vi "avaliaPresoNaParede.vi"(10 "Robot in":T3, 11 "IA State":T2={"our_robots"=[], "enemy_robots"=[], "balls"=[], "geometry"={"field_length"=0, "field_width"=0, "goal_width"=0, "goal_depth"=0, "center_circle_radius"=0, "defense_width"=0, "defense_depth"=0, "free_kick_from_defense_dist"=0, "penalty_spot_from_field_line_dist"=0, "penalty_line_from_spot_dist"=0, "half_moon_depth"=0, "half_moon_width"=0}, "IA Judge"={"stage"="", "command"="", "our_goalie_id"=0.0, "enemy_goalie_id"=0.0, "command enum"=enum."Halt", "Time"=enum."Azul"}, "Received Timestamp"=timestamp(0 s since 1904-01-01), "Events"={"Touch"=FALSE, "id touch"=0.0, "Ball out of \nVision"=FALSE, "Ball inside \nGoalie area"=FALSE, "Robot not responding"=FALSE, "Robots responding status"=[1.0, 1.0, 1.0, 1.0, 1.0, 1.0], "Enemy Ball \nPossession"=FALSE, "Id ini Possession"=0.0, "Ball Possesion"=FALSE, "Id Possesion"=0.0, "Ball at\nour goal side"=FALSE, "Ball at\ntouchline"=FALSE, "Ball at\nenemy goal side"=FALSE}}) -> (2 "Parede":T1(ring), 3 "Preso na parede?":bool=TRUE)   [LabVIEW 2018]
uses:
  Intel/Functions Enum.ctl
  Intel/AttackerStates.ctl
  Path Planning/RRT/PathDest.ctl
  Path Planning/RRT/PathDests.ctl
  Core/AI Robot.ctl
  Core/AI Ball.ctl
  Core/Field Size.ctl
  Intel/Command Enum.ctl
  Core/AI Judge.ctl
  Util/Events/Events.ctl
  Core/AI Input.ctl
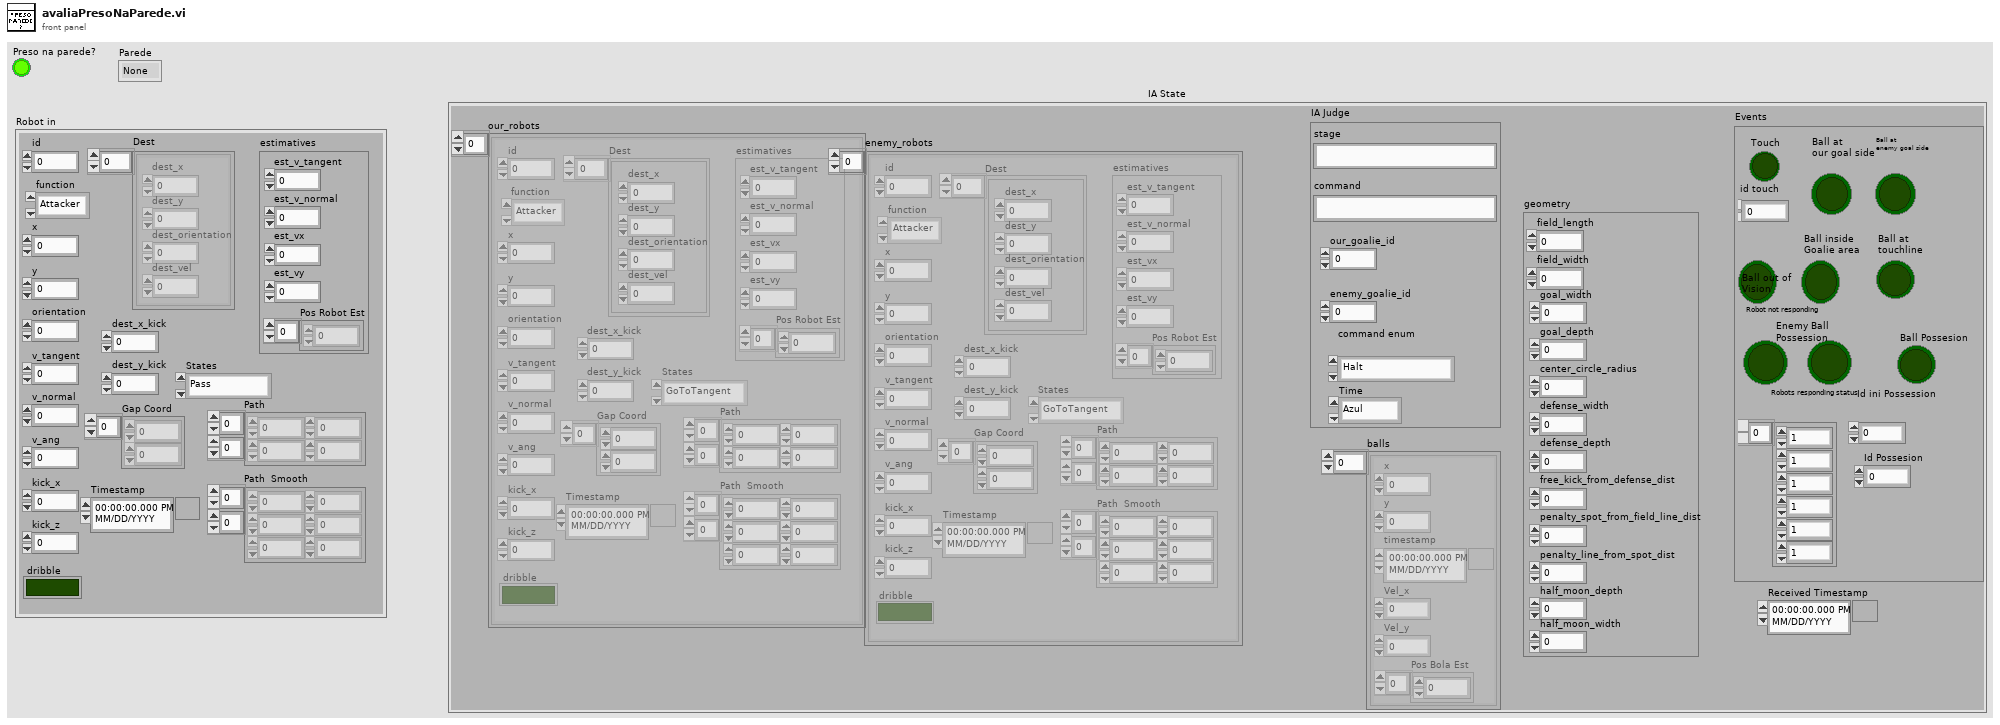
[diagram p1: front panel]
types:
  T1 = enum16{"None", "Frente", "Trás", "Cima", "Baixo"}
  T2 = typedef "AI Input.ctl" = cluster{"our_robots":T3[], "enemy_robots":T3[], "balls":T8[], "geometry":T9, "IA Judge":T10, "Received Timestamp":timestamp, "Events":T12}
  T3 = typedef "AI Robot.ctl" = cluster{"id":u32, "function":T4, "x":dbl, "y":dbl, "orientation":dbl, "v_tangent":dbl, "v_normal":dbl, "v_ang":dbl, "kick_x":dbl, "kick_z":dbl, "dribble":bool, "Timestamp":timestamp, "estimatives":cluster{"est_v_tangent":dbl, "est_v_normal":dbl, "est_vx":dbl, "est_vy":dbl, "Pos Robot Est":dbl[]}, "dest_x_kick":dbl, "dest_y_kick":dbl, "Gap Coord":dbl[], "States":T5, "Path ":dbl[][], "Path  Smooth":dbl[][], "Dest":T6}
  T4 = typedef "Functions Enum.ctl" = enum16{"Attacker", "Goalie", "Defender", "Striker", "Goto 0", "Dummy", "Kicker", "ZigZag"}
  T5 = typedef "AttackerStates.ctl" = enum16{"Pass", "GoToTangent", "BallGetting", "GoToKick", "Rotate anti-clockwise", "Rotate Clockwise", ""}
  T6 = typedef "PathDests.ctl" = T7[]
  T7 = typedef "PathDest.ctl" = cluster{"dest_x":dbl, "dest_y":dbl, "dest_orientation":dbl, "dest_vel":dbl}
  T8 = typedef "AI Ball.ctl" = cluster{"x":dbl, "y":dbl, "timestamp":timestamp, "Vel_x":dbl, "Vel_y":dbl, "Pos Bola Est":dbl[]}
  T9 = typedef "Field Size.ctl" = cluster{"field_length":u32, "field_width":u32, "goal_width":u32, "goal_depth":u32, "center_circle_radius":u32, "defense_width":u32, "defense_depth":u32, "free_kick_from_defense_dist":u32, "penalty_spot_from_field_line_dist":u32, "penalty_line_from_spot_dist":u32, "half_moon_depth":u32, "half_moon_width":u32}
  T10 = typedef "AI Judge.ctl" = cluster{"stage":string, "command":string, "our_goalie_id":dbl, "enemy_goalie_id":dbl, "command enum":T11, "Time":enum16{"Azul", "Amarelo"}}
  T11 = typedef "Command Enum.ctl" = enum16{"Halt", "Stop", "Force Start", "PKA Normal Start", "Prepare Kickoff Ally", "PKE Normal Start", "Prepare Kickoff Enemy", "Prepare Penalty Ally", "PPA Normal Start", "Prepare Penalty Enemy", "PPE Normal Start", "Ball Placement Enemy Up", "Ball Placement Enemy Down", "Ball Placement Ally Up", "Ball Placement Ally Mid", "Ball Placement Ally Down", "Indirect Free Enemy", "Indirect Free Ally", "Timeout Enemy", "Timeout Ally", "Goal Enemy", "Goal Ally", "Normal Half Time", "Extra Time Break", "Extra Half Time", "None", "Post Game"}
  T12 = typedef "Events.ctl" = cluster{"Touch":bool, "id touch":dbl, "Ball out of \nVision":bool, "Ball inside \nGoalie area":bool, "Robot not responding":bool, "Robots responding status":dbl[], "Enemy Ball \nPossession":bool, "Id ini Possession":dbl, "Ball Possesion":bool, "Id Possesion":dbl, "Ball at\nour goal side":bool, "Ball at\ntouchline":bool, "Ball at\nenemy goal side":bool}
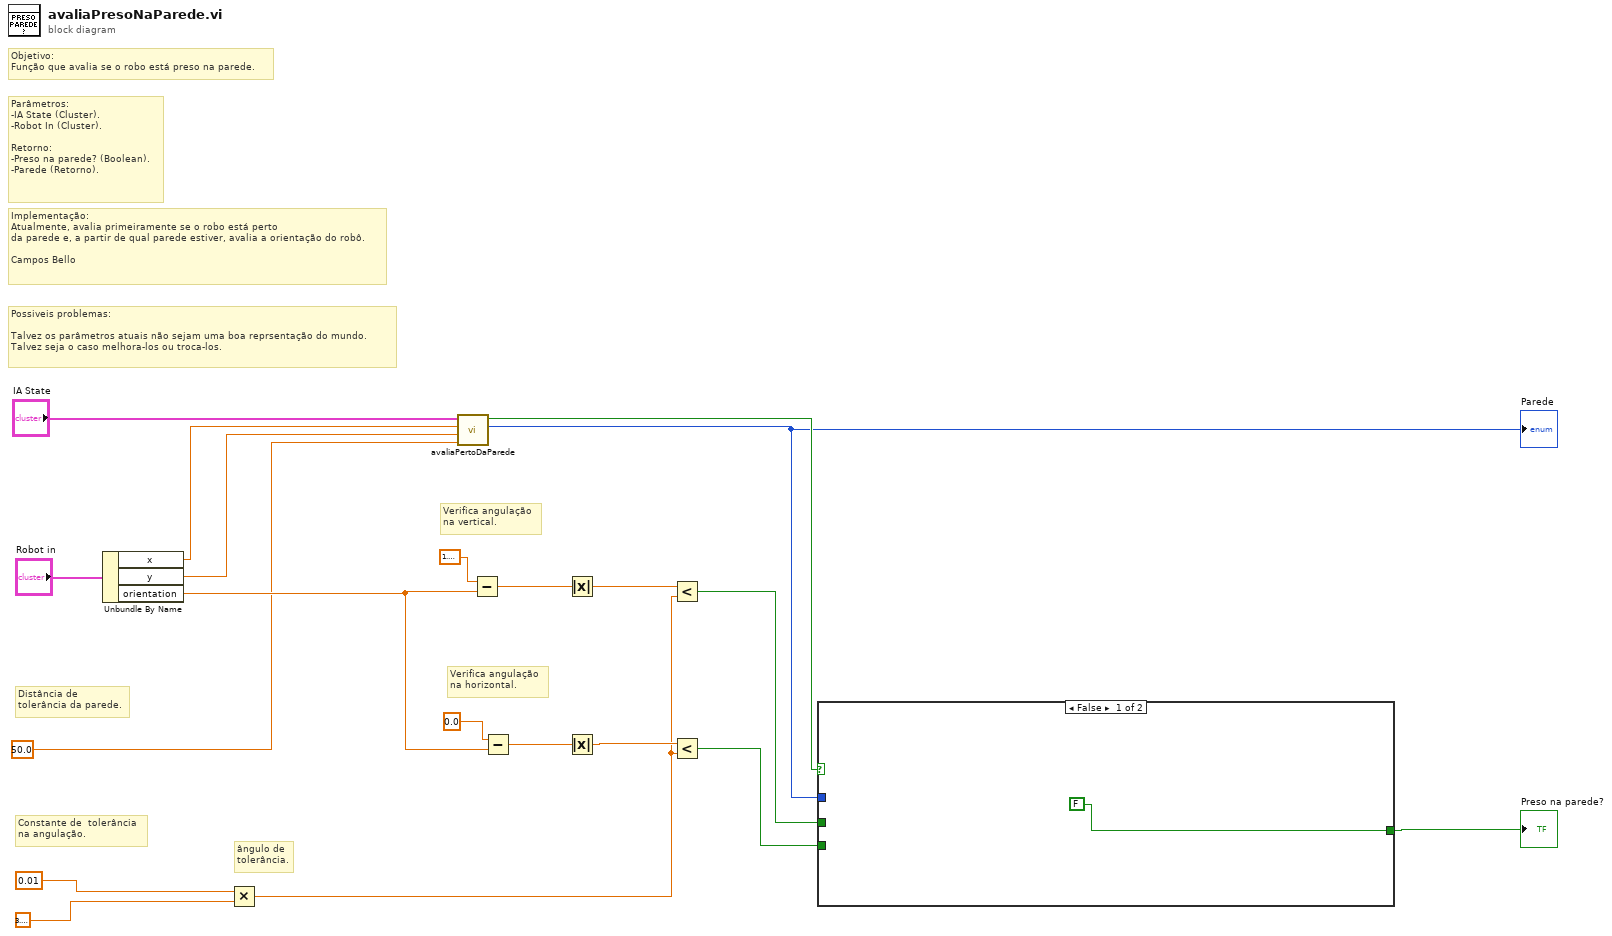
[diagram p0: block diagram]
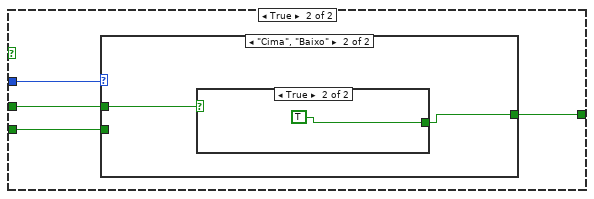
[diagram p2: hidden frame]
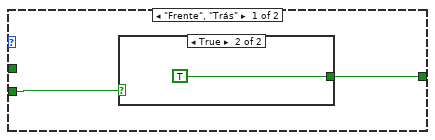
[diagram p3: hidden frame]
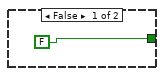
[diagram p4: hidden frame]
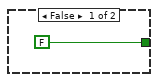
[diagram p5: hidden frame]
diagram:
  # "Possiveis problemas:\n\nTalvez os parâmetros atuais não sejam uma boa reprsentação do mundo.\nTalvez seja o caso melhora-los ou troca-los."
  # "Implementação:\nAtualmente, avalia primeiramente se o robo está perto\nda parede e, a partir de qual parede estiver, avalia a orientação do robô.\n\nCampos Bello"
  # "Parâmetros:\n-IA State (Cluster).\n-Robot In (Cluster).\n\nRetorno:\n-Preso na parede? (Boolean).\n-Parede (Retorno)."
  # "Objetivo:\nFunção que avalia se o robo está preso na parede."
  # "Distância de\ntolerância da parede."
  # "Verifica angulação\nna horizontal."
  # "Verifica angulação\nna vertical."
  # "ângulo de\ntolerância."
  # "Constante de  tolerância\nna angulação."
  n1 = Unbundle By Name("Robot in") -> ("x"=w8:dbl, "y"=w7:dbl, "orientation"=w15:dbl)
  n2 = Multiply(x=0.01, y=3.141592653589793) -> (x*y=w10:dbl)
  n3 = call "avaliaPertoDaParede.vi"("Distância"=50.0, "Y"=w7, "X"=w8, "IA State"="IA State") -> ("Enum"=w4:T1, "Perto de parede?"=w5:bool)  [unwired: 6 in]
  "Parede" <- w4
  n4 = Subtract(x=1.5707963267948966, y=w15) -> (x-y=w14:dbl)
  n5 = Subtract(x=0.0, y=w15) -> (x-y=w13:dbl)
  n6 = Absolute Value(x=w14) -> (abs(x)=w12:dbl)
  n7 = Absolute Value(x=w13) -> (abs(x)=w11:dbl)
  n8 = Less?(x=w12, y=w10) -> (x < y?=w3:bool)
  n9 = Less?(x=w11, y=w10) -> (x < y?=w2:bool)
  n10 = case shown="False" w5 {
    tunnel: w4 -> [_ w25]
    tunnel: w3 -> [_ w24]
    tunnel: w2 -> [_ w23]
    tunnel: [FALSE w22] -> w1
    frame False {
    }
    frame True {
      n11 = case shown="\"Cima\", \"Baixo\"" w25 {
        tunnel: w24 -> [_ w31]
        tunnel: w23 -> [w27 _]
        tunnel: [w26 w30] -> w22
        frame "Frente", "Trás" {
          n12 = case shown="True" w27 {
            tunnel: [FALSE TRUE] -> w26
            frame False {
            }
            frame True {
            }
          }
        }
        frame "Cima", "Baixo" {
          n13 = case shown="True" w31 {
            tunnel: [FALSE TRUE] -> w30
            frame False {
            }
            frame True {
            }
          }
        }
      }
    }
  }
  "Preso na parede?" <- w1
